vi "Process.vi"(8 "error in":errorcluster, 11 "Instrument UI.Transport":refnum<class "Inst UI.Transport.lvclass">) -> (0 "error out":errorcluster, 3 "Instrument UI.Transport out":refnum<class "Inst UI.Transport.lvclass">)   [LabVIEW 2019, in "Inst UI.Transport.lvclass"]
doc: "---------------------------------------------------------------\nJKI State Machine Objects™\nhttp://jki.net/state-machine-objects/\nCopyright (C) 2005-2015, JKI <info@jki.net>\nALL RIGHTS RESERVEDJKI State Machine Objects (SMO) 1.0.0.5\nJKI - JKI\nCopyright (c) 2016, JKI"
uses:
  Inst UI.Transport.lvclass
  C:/Program Files/National Instruments/LabVIEW 2019/vi.lib/JKI/JKI SMO/SMO/SMO.lvclass
  C:/Program Files/National Instruments/LabVIEW 2019/user.lib/LevyLab/Instrument Framework/Instrument UI/Instrument UI.lvclass
  C:/Program Files/National Instruments/LabVIEW 2019/vi.lib/JKI/JKI SMO/SMO.UI/SMO.UI.lvclass
  Inst.Transport/Typedefs/Inst.Transport.getAll--Cluster.ctl
  Inst.Transport/Inst.Transport.lvclass
  C:/Program Files/National Instruments/LabVIEW 2019/user.lib/LevyLab/Instrument Framework/Instrument/Instrument.lvclass
  Instrument UI.Transport.UI--Cluster.ctl
  Inst.Transport/Typedefs/Inst.Transport.Configuration--Cluster.ctl
  Transport/Typedefs/Lockin_Sweep JSON--Cluster.ctl
  <userlib>/LevyLab/Lockin-Multichannel/Instrument.DAQ/Typedefs/Sweep.Channel--Cluster--Array.ctl
  <userlib>/LevyLab/Lockin-Multichannel/Instrument.DAQ/Typedefs/Sweep.Channel--Cluster.ctl
  <userlib>/LevyLab/Lockin-Multichannel/Instrument.DAQ/Typedefs/Sweep.Pattern--Enum.ctl
  <userlib>/LevyLab/Configuration/Configuration.lvclass
  <userlib>/LevyLab/Instrument Framework/Instrument UI/Instrument UI.lvclass/Instrument UI.ctl
  <vilib>/JKI/JKI SMO/SMO/SMO.lvclass/SMO.ctl
  <userlib>/LevyLab/Configuration/Configuration.lvclass/Configuration.ctl
  2c224a34-a253-4174-b18d-44043a318d1a.vi
  <vilib>/dlg_ctls.llb/Space Constant.vi
  <vilib>/AdvancedString/1D String Array to Delimited String.vi
  <vilib>/JKI/JKI SMO/SMO/Private/ReftoDVR--SMO.vi
  2c224a34-a253-4174-b18d-44043a318d1a.vi/26bc7fe7-399c-42c0-9e9a-60ca208975aa.vi
  2c224a34-a253-4174-b18d-44043a318d1a.vi/9995e869-8f6f-46da-9c29-74663bf4c27c.vi
  <vilib>/Utility/Data Type/Get Type Information.vi
  <vilib>/JDP Science/JSONtext/JSON text to Variant.vi
  <userlib>/LevyLab/Instrument Framework/Instrument/Instrument.lvclass
  <vilib>/JDP Science/JSONtext/LVClass Serializer/JSONtext LVClass Serializer.lvclass
  <userlib>/LevyLab/Instrument Framework/Instrument UI/Instrument UI.lvclass
  <userlib>/LevyLab/Debug/Debug.lvlib
  <vilib>/JKI/JKI SMO/SMO/SMO.lvclass
  <vilib>/JKI/JKI SMO/SMO.UI/SMO.UI.lvclass
  <userlib>/LevyLab/Lockin-Multichannel/Instrument.DAQ/Instrument.DAQ.lvclass
  Transport/Transport.lvclass
panel:
  out "Secret Status":string
  out "State History":string
  in  "STOP":bool
  # "Transport Server"
  # "SMO UI Template"
  # "For instructions on how to use the JKI State Machine Objects, examples and video tutorials, visit:\nhttp://jki.net/state-machine-objects/\n\nJKI State Machine Objects™\nhttp://jki.net/state-machine-objects/\nCopyright (C) 2005-2015, JKI <info@jki.net>\nALL RIGHTS RESERVED"
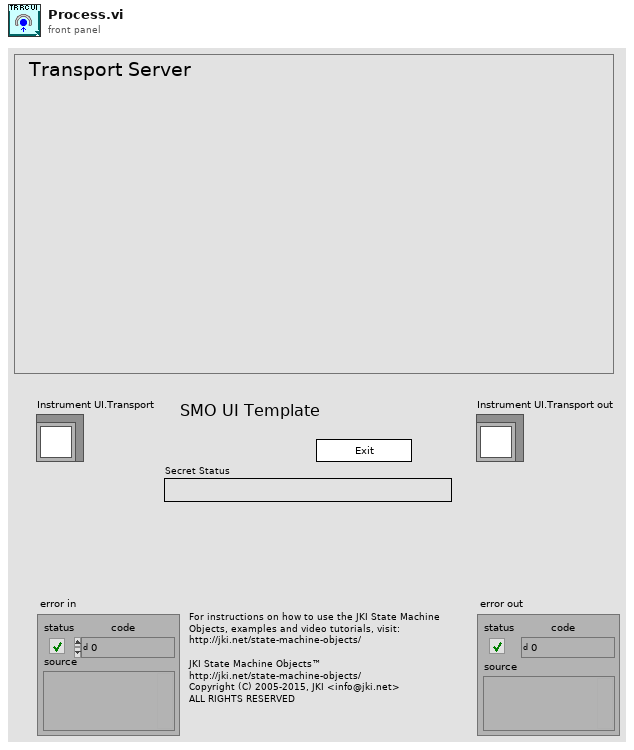
[diagram p1: front panel]
types:
  T1 = enum32{"invalid app kind", "Development System", "Run Time System", "Student Edition", "Embedded LabVIEW", "Evaluation", "Custom"}
  T2 = enum32{"Invalid", "Standard", "Closed", "Hidden", "Minimized", "Maximized"}
  T3 = typedef "Inst.Transport.lvclass/Inst.Transport.Configuration--Cluster.ctl" = cluster{"Folder":string, "Comments":string, "Sweep":T4}
  T4 = typedef "Transport.lvclass/Lockin_Sweep JSON--Cluster.ctl" = cluster{"initialWaitTime":dbl, "sweepTime":dbl, "Return to Start":bool, "sweepChannels":T5, "sweepTables":cluster{"Ch":i32, "Table":dbl[]}[]}
  T5 = typedef "Instrument.Lockin.lvlib/Instrument.DAQ.lvclass/Sweep.Channel--Cluster--Array.ctl" = T6[]
  T6 = typedef "Instrument.Lockin.lvlib/Instrument.DAQ.lvclass/Sweep.Channel--Cluster.ctl" = cluster{"Enable?":bool, "Channel":u16, "Start":dbl, "End":dbl, "Pattern":T7, "Table":dbl[]}
  T7 = typedef "Instrument.Lockin.lvlib/Instrument.DAQ.lvclass/Sweep.Pattern--Enum.ctl" = enum16{"Ramp /", "Ramp /\\", "Smooth Ramp _/", "Smooth Ramp _/\\_", "Table"}
  T8 = typedef "Inst.Transport.lvclass/Inst.Transport.getAll--Cluster.ctl" = cluster{"data":variant}
  T9 = typedef "Inst UI.Transport.lvclass/Instrument UI.Transport.UI--Cluster.ctl" = cluster{"Parameter":dbl, "Parameter 2":string}
  T10 = cluster{"Core":cluster{"Current VI Reference":refnum<vi>, "Close Panel on Exit?":bool, "Last Error":cluster{"error":errorcluster, "previous state":string, "remaining states":string}, "Shutdown?":bool}, "Instrument UI":refnum<class "Inst UI.Transport.lvclass">, "Instrument":refnum<class "Inst.Transport.lvclass">, "Configuration":refnum<class "Configuration.lvclass">, "Config Cluster":T3, "getAll":T8, "UI Cluster":T9, "UI Behavior":string, "wait":u32}
  T11 = cluster{"Current VI Reference":refnum<vi>, "Close Panel on Exit?":bool, "Last Error":cluster{"error":errorcluster, "previous state":string, "remaining states":string}, "Shutdown?":bool}
  T12 = typedef "Debug.lvlib/Attribute.Debug.lvclass/DebugBehavior.ctl" = enum16{"Normal", "Debug"}
  T13 = typedef "SMO.lvclass/Protected Events.ctl" = cluster{"StopProcesses":refnum<user-event>, "AbortProcesses":refnum<user-event>, "Config Changed":refnum<user-event>, "Dependency":refnum<user-event>}
  T14 = typedef "Instrument.lvlib/Instrument.lvclass/PublicEvents--Cluster.ctl" = cluster{"MessageFromProcess":refnum<user-event>}
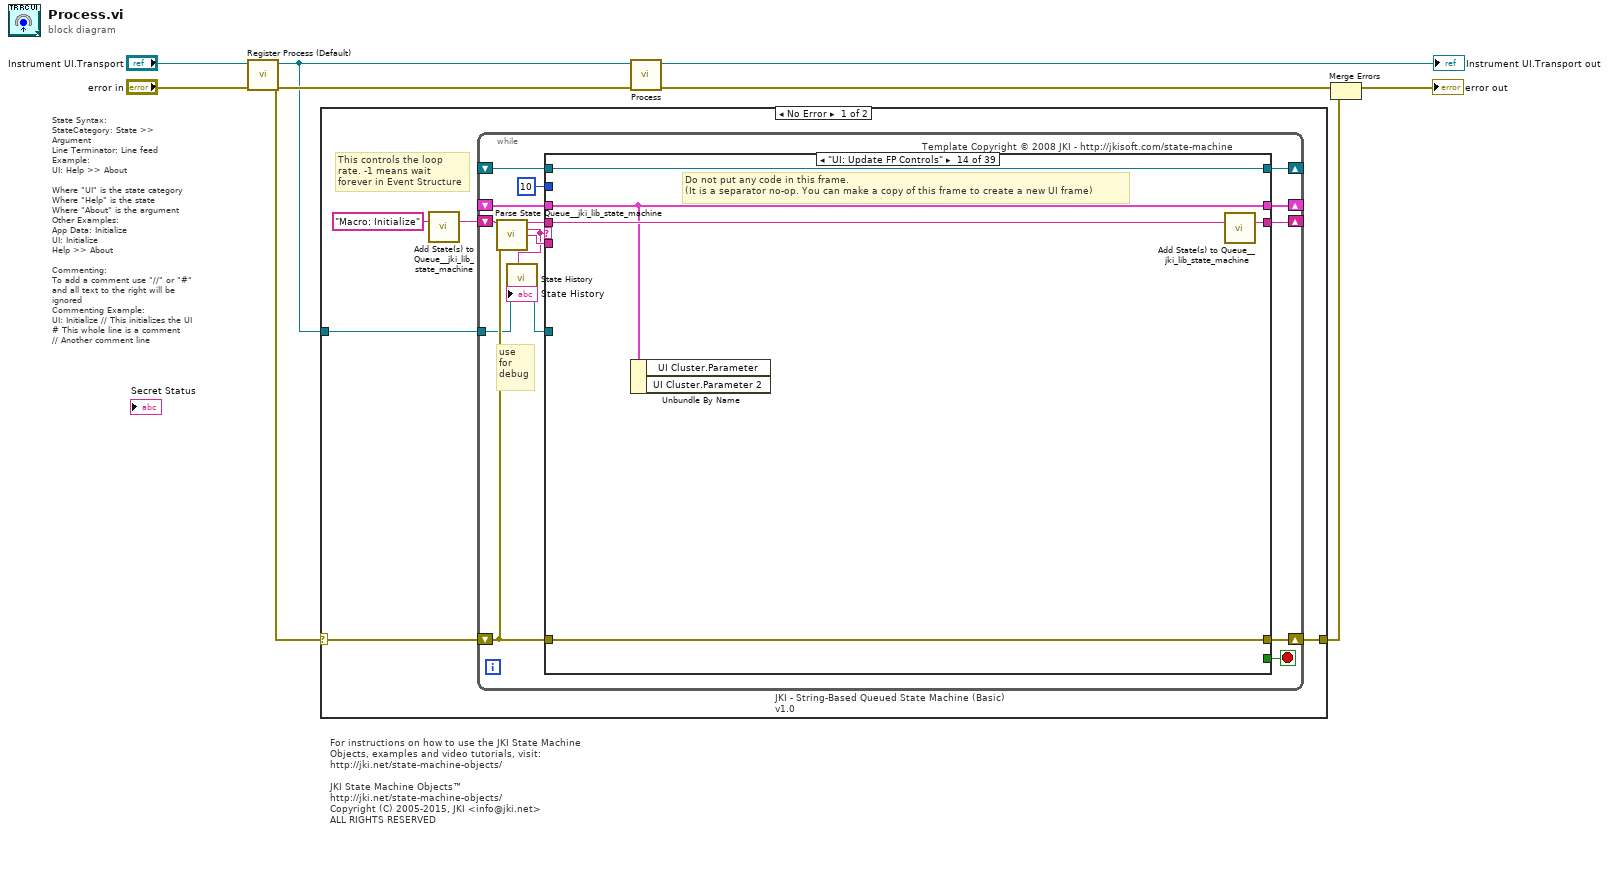
[diagram p0: block diagram]
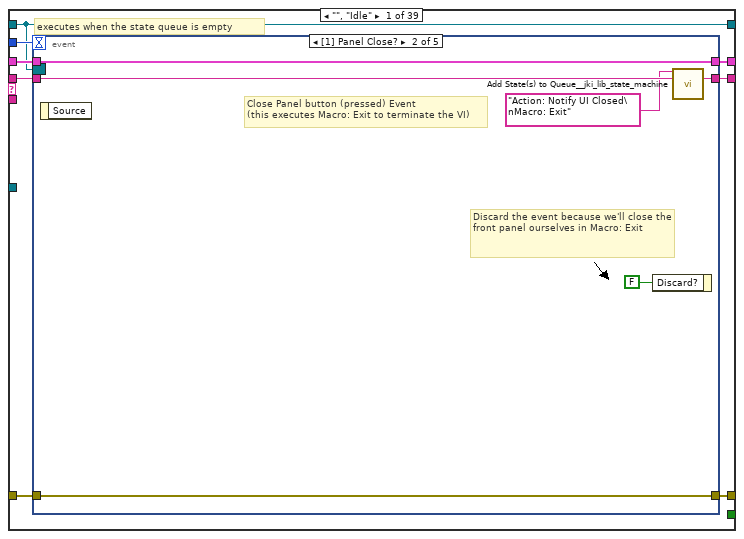
[diagram p2: hidden frame]
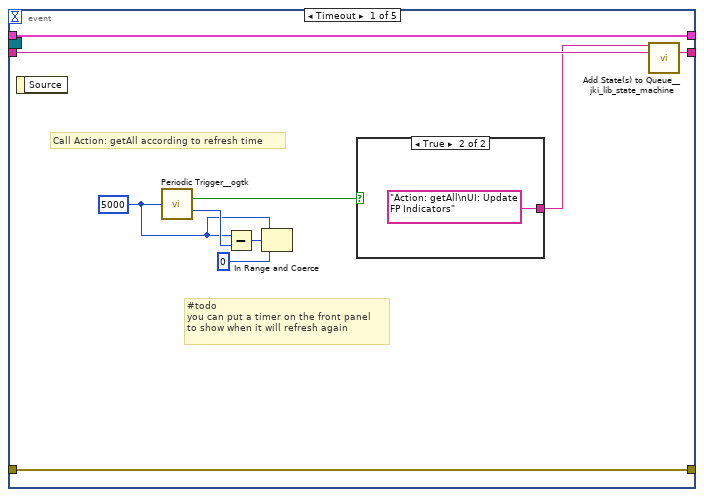
[diagram p3: hidden frame]
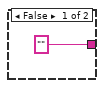
[diagram p4: hidden frame]
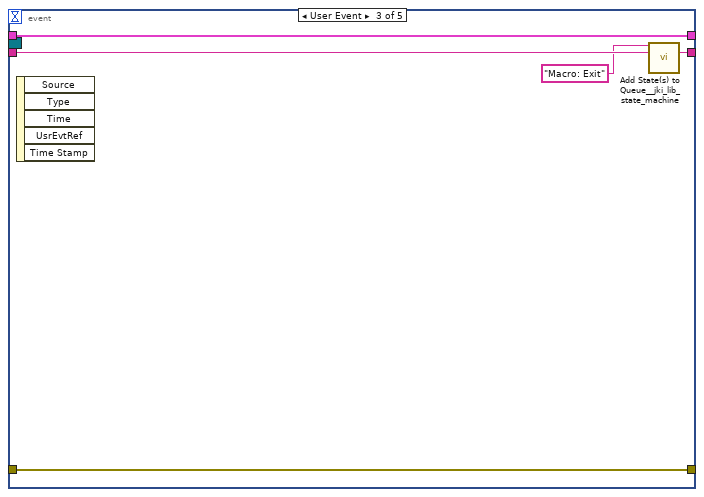
[diagram p5: hidden frame]
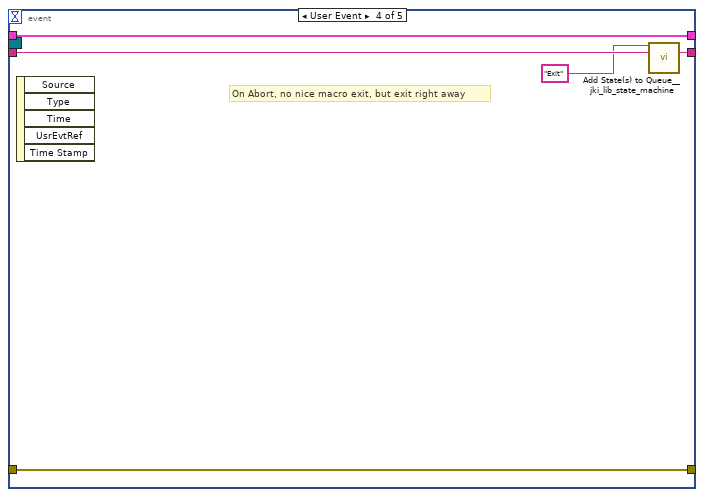
[diagram p6: hidden frame]
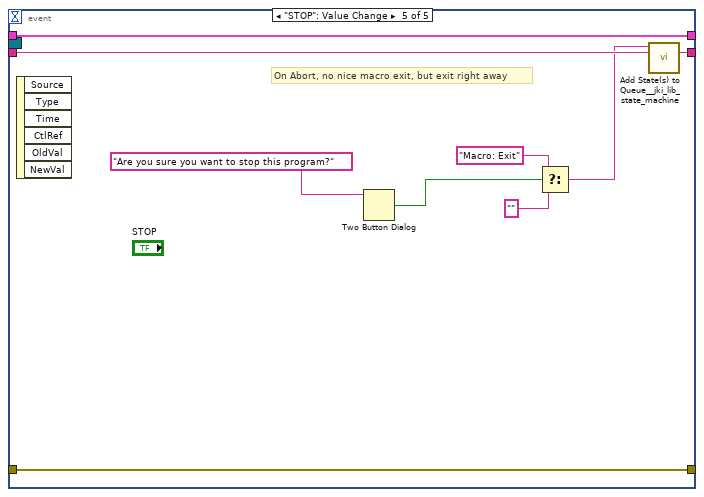
[diagram p7: hidden frame]
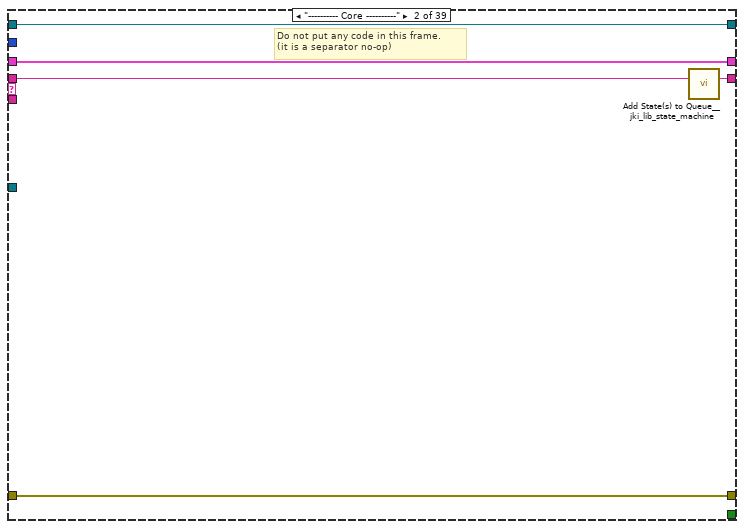
[diagram p8: hidden frame]
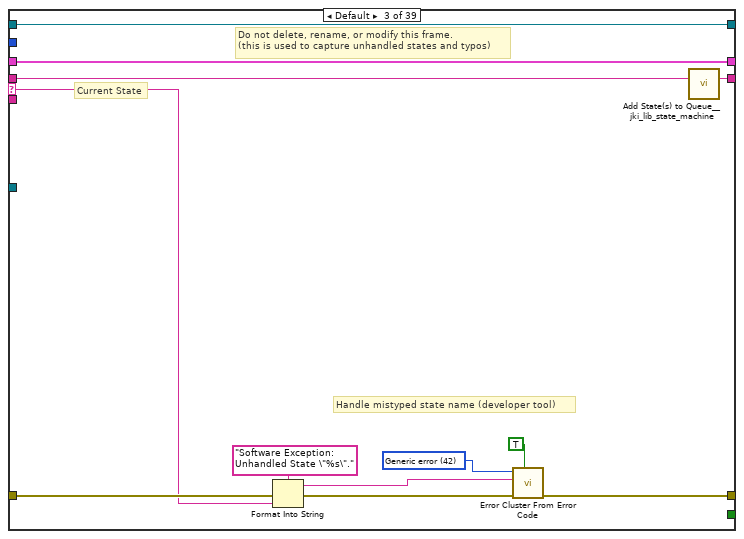
[diagram p9: hidden frame]
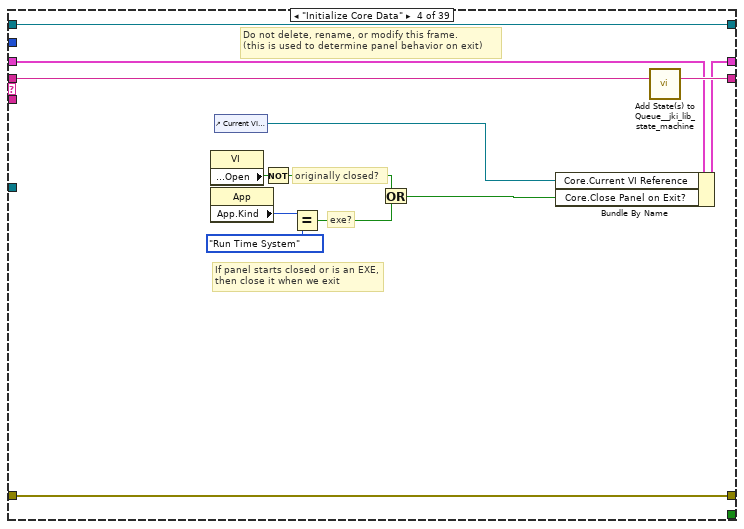
[diagram p10: hidden frame]
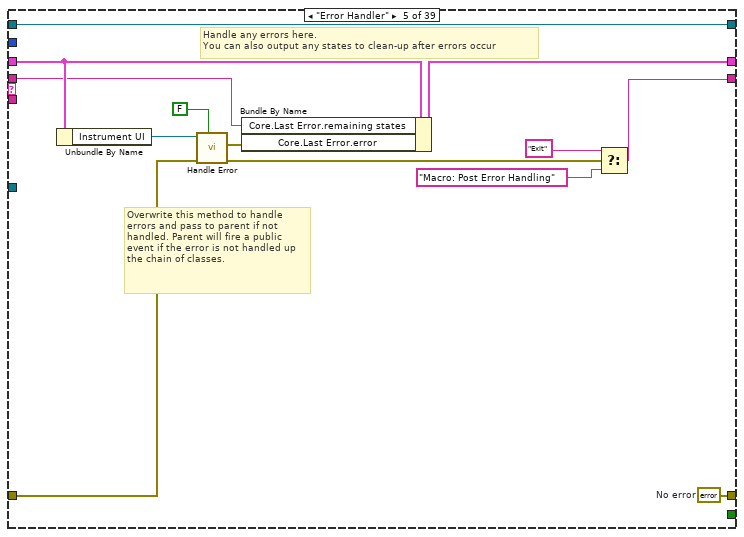
[diagram p11: hidden frame]
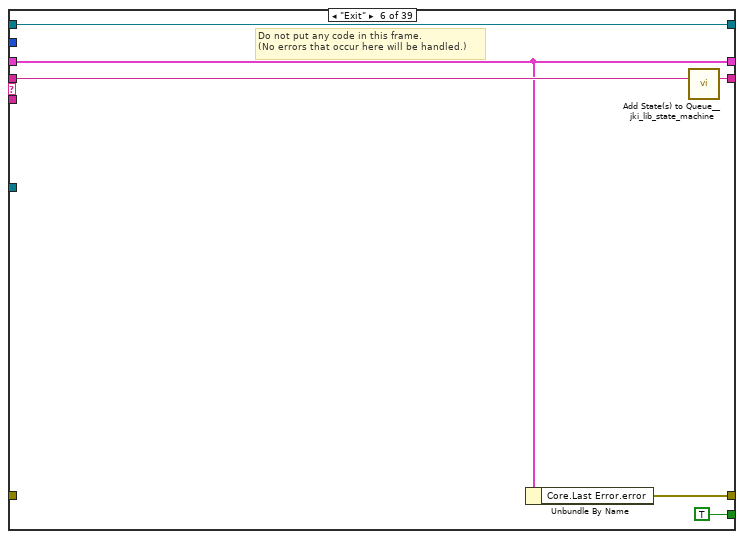
[diagram p12: hidden frame]
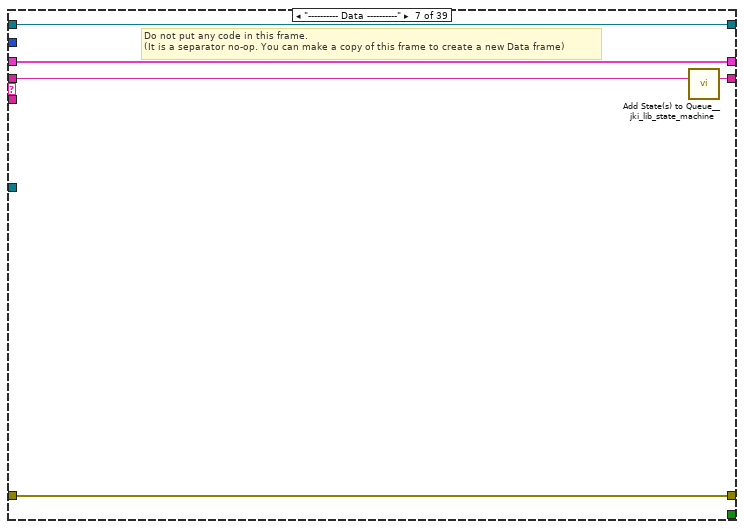
[diagram p13: hidden frame]
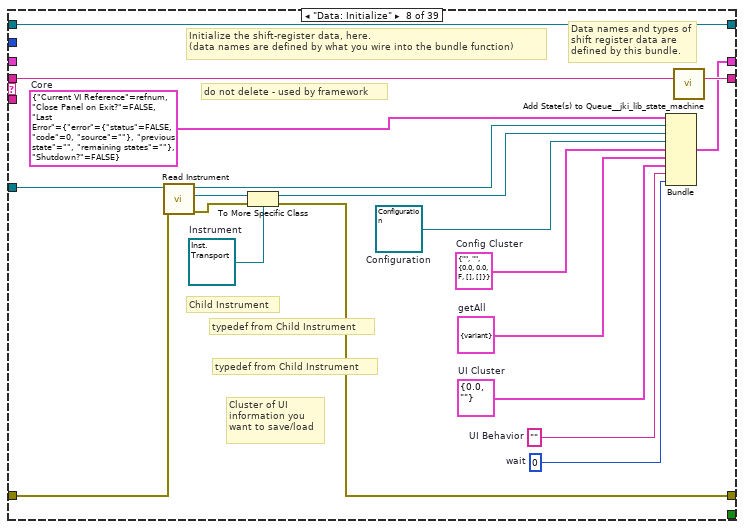
[diagram p14: hidden frame]
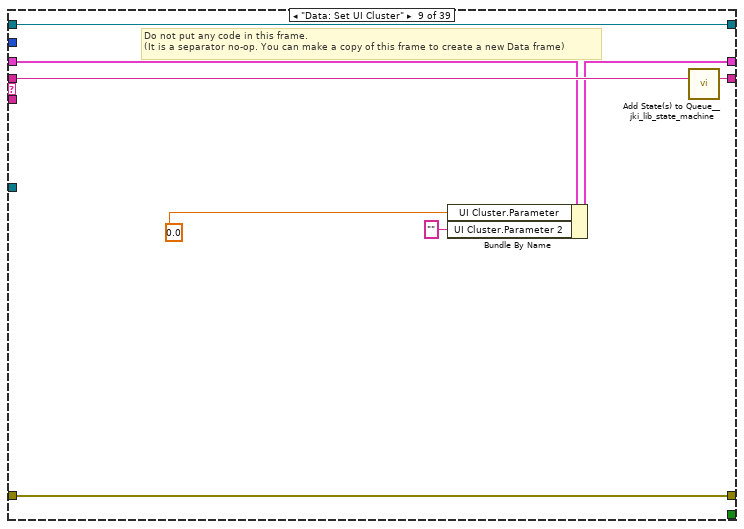
[diagram p15: hidden frame]
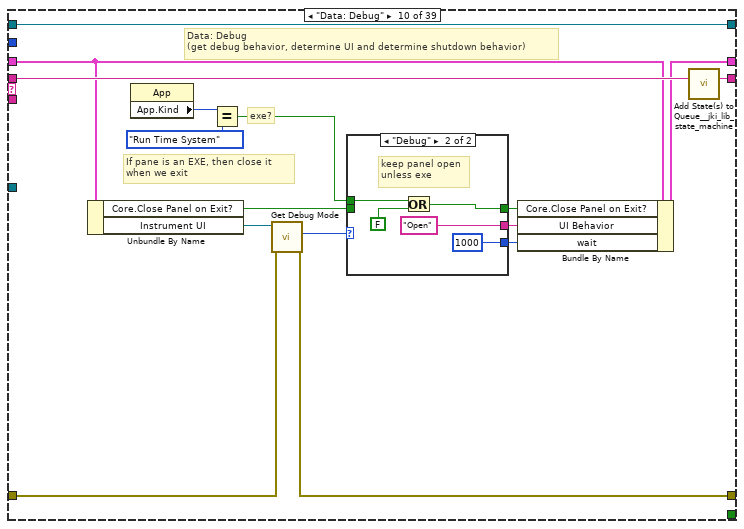
[diagram p16: hidden frame]
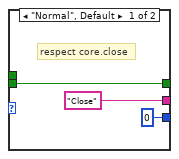
[diagram p17: hidden frame]
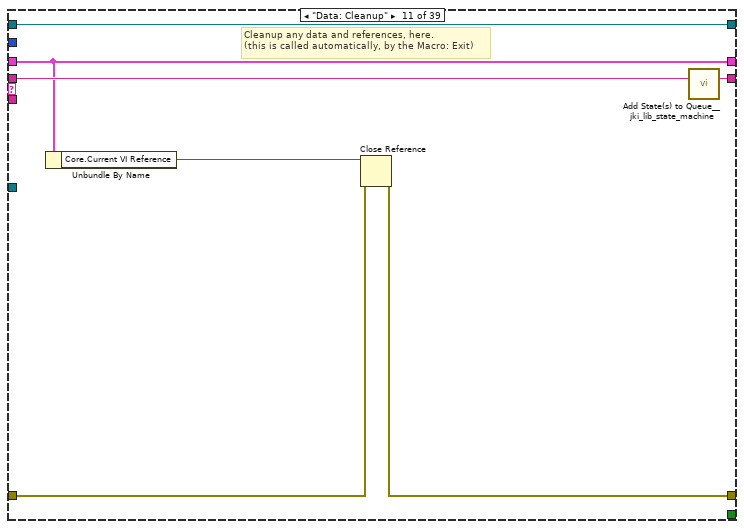
[diagram p18: hidden frame]
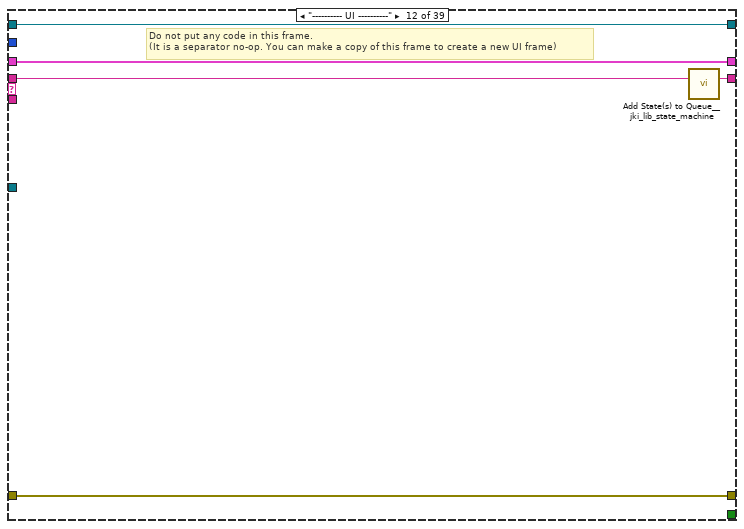
[diagram p19: hidden frame]
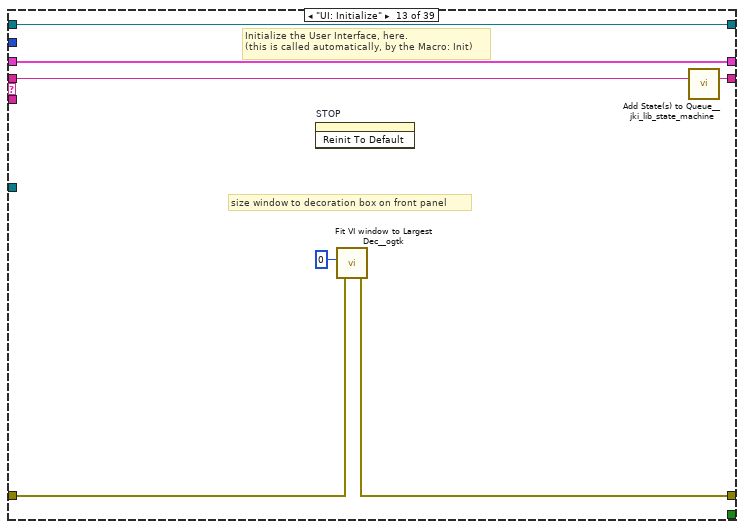
[diagram p20: hidden frame]
diagram:
  # "State Syntax:\nStateCategory: State >> Argument\nLine Terminator: Line feed\nExample:\nUI: Help >> About\n\nWhere \"UI\" is the state category\nWhere \"Help\" is the state\nWhere \"About\" is the argument\nOther Examples:\nApp Data: Initialize\nUI: Initialize\nHelp >> About\n\nCommenting:\nTo add a comment use \"//\" or \"#\" and all text to the right will be ignored\nCommenting Example:\nUI: Initialize // This initializes the UI\n# This whole line is a comment\n// Another comment line"
  # "For instructions on how to use the JKI State Machine Objects, examples and video tutorials, visit:\nhttp://jki.net/state-machine-objects/\n\nJKI State Machine Objects™\nhttp://jki.net/state-machine-objects/\nCopyright (C) 2005-2015, JKI <info@jki.net>\nALL RIGHTS RESERVED"
  n1 = call <vilib>:"Register Process (Default).vi"("error in (no error)"="error in", "SMO"="Instrument UI.Transport") -> ("error out"=w5:errorcluster, "SelfRef"=w4:refnum<class "Inst UI.Transport.lvclass">)  [unwired: 8 in]
  n2 = case shown="No Error" w5 {
    selector: w5 -> [w10 w459]
    tunnel: w4 -> [w11 _]
    tunnel: [w9 w459] -> w1
    frame No Error {
      # "This controls the loop rate. -1 means wait forever in Event Structure"
      n3 = call <vilib>:"Add State(s) to Queue__jki_lib_state_machine.vi"("State(s) in (\"\")"="Macro: Initialize") -> ("States Out"=w13:string)  [unwired: 14 in]
      n4 = while "JKI - String-Based Queued State Machine (Basic) v1.0" {
        shift-right: [w23] -> _
        shift-left: _ -> [w22]
        shift-right: [w26] -> w9
        shift-left: w10 -> [w18]
        shift-right: [w25] -> _
        shift-left: w13 -> [w27]
        tunnel: w11 -> [w14]
        shift-right: [w20] -> _
        shift-left: _ -> [w19]
        stop <- w24 stop-if-true
        # "use\nfor\ndebug"
        # "Template Copyright © 2008 JKI - http://jkisoft.com/state-machine"
        n5 = call <vilib>:"Parse State Queue__jki_lib_state_machine.vi"("State Queue"=w27, "Error In (no error)"=w18) -> ("Remaining States"=w29:string, "Current State"=w17:string, "Arguments"=w28:string)  [unwired: 11 in]
        n6 = call <userlib>:"State History.vi"("Current State"=w17, "SMO"=w14) -> ("SMO"=w15:refnum<class "Inst UI.Transport.lvclass">, "History"=→"State History":string)  [unwired: 8 in]
        n7 = case shown="\"UI: Update FP Controls\"" w17 {
          selector: w17 -> [_ _ w81 _ _ _ _ _ _ _ _ _ _ _ _ _ _ _ _ _ _ _ _ _ _ _ _ _ _ _ _ _ _ _ _ _ _ _ _]
          tunnel: w29 -> [w37 w79 w85 w104 w108 w123 w128 w147 w155 w171 w186 w191 w198 w203 w208 w215 w231 w263 w272 w284 w294 w300 w308 w323 w328 w339 w346 w351 w364 w370 w375 w390 w398 w410 w417 w424 w438 w448 w458]
          tunnel: w28 -> [_ _ _ _ _ _ _ _ _ _ _ _ _ _ _ w209 w225 _ _ _ _ _ _ _ _ _ _ _ _ _ _ _ _ _ _ _ _ _ _]
          tunnel: w22 -> [w35 w76 w83 w95 w111 w119 w125 _ w151 w158 w180 w188 w196 w199 w204 w213 w227 w260 w269 w274 w291 w297 w302 w312 w325 w336 w341 w348 w362 w368 w372 w383 w395 w401 w413 w418 w433 w442 w450]
          tunnel: [w34 w77 w87 w101 w113 w118 w126 w129 w153 w157 w182 w189 w193 w201 w205 w210 w228 w261 w264 w282 w292 w298 w306 w321 w326 w330 w342 w349 w357 w365 w373 w376 w393 w402 w414 w419 w431 w445 w455] -> w26
          tunnel: [w36 w78 w84 w103 w105 w122 w127 w146 w154 w170 w185 w190 w197 w202 w207 w214 w230 w262 w271 w283 w293 w299 w307 w322 w327 w338 w345 w350 w363 w369 w374 w389 w397 w409 w416 w423 w437 w447 w457] -> w25
          tunnel: [_ _ _ _ _ TRUE _ _ _ _ _ _ _ _ _ _ _ _ _ _ _ _ _ _ _ _ _ _ _ _ _ _ _ _ _ _ _ _ _] -> w24
          tunnel: [w32 w76 w83 w102 w110 w119 w125 w145 w150 w159 w180 w188 w196 w199 w204 w213 w227 w260 w269 w275 w291 w297 w302 w312 w325 w336 w341 w348 w362 w368 w372 w387 w395 w399 w412 w418 w434 w443 w452] -> w23
          tunnel: 10 ("Timeout") -> [w31 _ _ _ _ _ _ _ _ _ _ _ _ _ _ _ _ _ _ _ _ _ _ _ _ _ _ _ _ _ _ _ _ _ _ _ _ _ _]
          tunnel: w15 -> [_ _ _ _ _ _ _ w134 _ _ _ _ _ _ _ _ _ _ _ _ _ _ _ _ _ _ _ _ _ _ _ _ _ _ _ _ _ _ _]
          tunnel: [w30 w75 w80 w92 w117 w120 w124 w144 w152 w169 w181 w187 w195 w200 w206 w212 w224 w259 w270 w281 w290 w296 w305 w317 w324 w337 w344 w347 w361 w367 w371 w388 w396 w408 w415 w422 w436 w446 w456] -> w20
          tunnel: w19 -> [w30 w75 w80 w92 w117 w120 w124 w144 w152 w169 w181 w187 w195 w200 w206 w212 w224 w259 w270 w281 w290 w296 w305 w317 w324 w337 w344 w347 _ w367 w371 w388 w396 w408 w415 w422 w436 w446 w456]
          tunnel: w18 -> [w33 w77 w86 w101 w107 _ w126 w133 w153 w156 w183 w189 w194 w201 w205 w211 w229 w261 w264 w282 w292 w298 w306 w321 w326 w331 w343 w349 w359 w366 w373 w385 w391 w403 w414 w420 w425 w439 w451]
          frame "", "Idle" {
            # "executes when the state queue is empty"
            n8 = event shown="[1] Panel Close?" {
              selector: w30 -> [_ _ _ _ _]
              dyn-events: _ -> [_ _ _ _ _]
              timeout: w31 -> [_ _ _ _ _]
              tunnel: w37 -> [w47 w55 w60 w65 w74]
              tunnel: [w46 w54 w59 w64 w73] -> w36
              tunnel: w35 -> [w44 w51 w57 w62 w71]
              tunnel: [w45 w50 w58 w63 w72] -> w34
              tunnel: w33 -> [w45 w50 w58 w63 w72]
              tunnel: [w44 w51 w57 w62 w71] -> w32
              event Timeout {
                w39 = u32 5000 ("time (ms)")
                # "#todo\nyou can put a timer on the front panel\nto show when it will refresh again"
                # "Call Action: getAll according to refresh time"
                n9 = event-data() -> ()  [unwired: 1 in, 1 out]
                n10 = call <userlib>:"Periodic Trigger__ogtk.vi"("time (ms)"=w39) -> ("Triggered"=w42:bool, "timer value"=w41:u32)  [unwired: 12 in, 1 out]
                n11 = Subtract(x=w39, y=w41) -> (x-y=w40:u32)
                n12 = In Range and Coerce(upper limit=w39, x=w40, lower limit=u32 0) -> ()  [unwired: 2 out]
                n13 = case shown="True" w42 {
                  tunnel: ["" ("State(s) in Front (\"\")") "Action: getAll\nUI: Update FP Indicators" ("State(s) in Front (\"\")")] -> w43
                  frame False {
                  }
                  frame True {
                  }
                }
                n14 = call <vilib>:"Add State(s) to Queue__jki_lib_state_machine.vi"("State(s) in Front (\"\")"=w43, "State(s) in (\"\")"=w47) -> ("States Out"=w46:string)  [unwired: 13 in]
              }
              event Panel Close? {
                # "Discard the event because we'll close the front panel ourselves in Macro: Exit"
                # "Close Panel button (pressed) Event\n(this executes Macro: Exit to terminate the VI)"
                n15 = event-data() -> ()  [unwired: 1 in, 1 out]
                n16 = event-data("Discard?"=FALSE) -> ()  [unwired: 1 in, 1 out]
                n17 = call <vilib>:"Add State(s) to Queue__jki_lib_state_machine.vi"("State(s) in Front (\"\")"="Action: Notify UI Closed\nMacro: Exit", "State(s) in (\"\")"=w55) -> ("States Out"=w54:string)  [unwired: 13 in]
              }
              event User Event {
                n18 = event-data() -> ()  [unwired: 1 in, 5 out]
                n19 = call <vilib>:"Add State(s) to Queue__jki_lib_state_machine.vi"("State(s) in Front (\"\")"="Macro: Exit", "State(s) in (\"\")"=w60) -> ("States Out"=w59:string)  [unwired: 13 in]
              }
              event User Event {
                # "On Abort, no nice macro exit, but exit right away"
                n20 = event-data() -> ()  [unwired: 1 in, 5 out]
                n21 = call <vilib>:"Add State(s) to Queue__jki_lib_state_machine.vi"("State(s) in Front (\"\")"="Exit", "State(s) in (\"\")"=w65) -> ("States Out"=w64:string)  [unwired: 13 in]
              }
              event "STOP": Value Change {
                # "On Abort, no nice macro exit, but exit right away"
                n22 = event-data() -> ()  [unwired: 1 in, 6 out]
                n23 = Two Button Dialog(message="Are you sure you want to stop this program?") -> (T button?=w70:bool)  [unwired: 2 in]
                n24 = Select(t="Macro: Exit", s=w70, f="") -> (s? t:f=w66:string)
                n25 = call <vilib>:"Add State(s) to Queue__jki_lib_state_machine.vi"("State(s) in Front (\"\")"=w66, "State(s) in (\"\")"=w74) -> ("States Out"=w73:string)  [unwired: 13 in]
              }
            }
          }
          frame "---------- Core ----------" {
            # "Do not put any code in this frame.\n(it is a separator no-op)"
            n26 = call <vilib>:"Add State(s) to Queue__jki_lib_state_machine.vi"("State(s) in (\"\")"=w79) -> ("States Out"=w78:string)  [unwired: 14 in]
          }
          frame Default {
            w90 = 42 items=["No error", "Argument error", "Memory is full", "Out of zone", "End of file", "File already open", "Generic file I/O error", "File not found", "File permission error", "Disk is full", "Duplicate path", "Too many files open", "System feature not enabled", "Resource file not found", "Cannot add resource", "Resource not found", "Image not found", "Image memory error", "Pen does not exist", "Config type invalid", "Config token not found", "Config parse error", "Config memory error", "Bad external code format", "Bad external code offset", "External code not present", "Null window", "Destroy window error", "Null menu", "Print aborted", "Bad print record", "Print driver error", "Windows error during printing", "Memory error during printing", "Print dialog error", "Generic print error", "Invalid device refnum", "Device not found", "Device parameter error", "Device unit error", "Cannot open device", "Device call aborted", "Generic error", "Cancelled by user", "Object ID too low", "Object ID too high", "Object not in heap", "Unknown heap", "Unknown object (invalid DefProc)", "Unknown object (DefProc not in table)", "Message out of range", "Invalid (null) method", "Unknown message", "Manager call not supported", "Bad address", "Network operation in progress", "Network operation timed out", "Connection is busy", "Network attribute not supported", "Network error", "Address in use", "System out of memory", "Connection aborted", "Connection refused", "Not connected", "Already connected", "Connection closed", "Initialization error (interapplication manager)", "Bad occurrence", "Wait on unbound occurrence handler", "Occurrence queue overflow", "Datalog type conflict", "Unused", "Unrecognized type (interapplication manager)", "Memory corrupt", "Failed to make temporary DLL", "Old CIN version", "Drag socket not found", "Failed to load drop-object", "Failed to register OLE object", "Failed to release OLE object", "Format specifier type mismatch", "Unknown format specifier", "Too few format specifiers", "Too many format specifiers", "Scan failed", "Newer CIN version", "Error converting to variant", "Runtime menu error", "Password tampered", "Variant attribute not found", "Incompatible variant data type", "Event data is not available", "Event Store is not present", "Occurrence is not found", "Event Queue is not created", "Event info is not available", "Refnum passed is NULL", "Error retrieving Class GUID", "Error retrieving CoClass GUID", "Error retrieving TypeLib GUID.", "Bad built application magic bytes.", "Specific driver is different from the specific driver associated with the Logical Name.", "There is no session opened to the class driver.", "Max Error", "MAX - Error with config objects", "MAX - Error loading configuration", "MAX - Group not supported"]
            # "Current State"
            # "Do not delete, rename, or modify this frame.\n(this is used to capture unhandled states and typos)"
            # "Handle mistyped state name (developer tool)"
            n27 = Format Into String(format string="Software Exception: Unhandled State \"%s\"." ("message"), error in=w86, w81) -> (resulting string=w89:string, error out=w88:errorcluster)  [unwired: 1 in]
            n28 = call <vilib>:"Error Cluster From Error Code.vi"("show call chain? (False)"=TRUE, "error in (no error)"=w88, "error message (\"\")"=w89, "error code (0)"=w90) -> ("error out"=w87:errorcluster)  [unwired: 5 in]
            n29 = call <vilib>:"Add State(s) to Queue__jki_lib_state_machine.vi"("State(s) in (\"\")"=w85) -> ("States Out"=w84:string)  [unwired: 14 in]
          }
          frame "Initialize Core Data" {
            # "Do not delete, rename, or modify this frame.\n(this is used to determine panel behavior on exit)"
            # "originally closed?"
            # "exe?"
            # "If panel starts closed or is an EXE, then close it when we exit"
            n30 = property class="VI"() -> ("Front Panel.Open"=w100:bool)  [unwired: 2 in, 2 out]
            n31 = property class="App"() -> ("App.Kind"=w99:T1)  [unwired: 2 in, 2 out]
            n32 = control-ref of="Current VI Reference"() -> (w93:refnum<vi>)
            n33 = Not(x=w100) -> (.not. x?=w97:bool)
            n34 = Equal?(x=w99, y=T1."Run Time System" ("Application:Kind")) -> (x = y?=w96:bool)
            n35 = Or(x=w97, y=w96) -> (x .or. y?=w94:bool)
            n36 = Bundle By Name(cluster=w95, "Core.Current VI Reference"=w93, "Core.Close Panel on Exit?"=w94) -> (w102:T10)
            n37 = call <vilib>:"Add State(s) to Queue__jki_lib_state_machine.vi"("State(s) in (\"\")"=w104) -> ("States Out"=w103:string)  [unwired: 14 in]
          }
          frame "Error Handler" {
            w113 = errorcluster {"status"=FALSE, "code"=0, "source"=""}  # No error
            # "Overwrite this method to handle errors and pass to parent if not handled. Parent will fire a public event if the error is not handled up the chain of classes."
            # "Handle any errors here.\nYou can also output any states to clean-up after errors occur"
            n38 = Unbundle By Name(w111) -> ("Instrument UI"=w116:refnum<class "Inst UI.Transport.lvclass">)
            n39 = call-dynamic "Handle Error.vi"("Stop on Unhandled Error (T)"=FALSE, "error in"=w107, "SMO"=w116) -> ("handling error"=w114:errorcluster, "Unhandled error"=w112:errorcluster)  [unwired: 6 in, 1 out]
            n40 = Bundle By Name(cluster=w111, "Core.Last Error.remaining states"=w108, "Core.Last Error.error"=w112) -> (w110:T10)
            n41 = Select(t="Exit", s=w114, f="Macro: Post Error Handling") -> (s? t:f=w105:string)
          }
          frame "Exit" {
            # "Do not put any code in this frame.\n(No errors that occur here will be handled.)"
            n42 = Unbundle By Name(w119) -> ("Core.Last Error.error"=w118:errorcluster)
            n43 = call <vilib>:"Add State(s) to Queue__jki_lib_state_machine.vi"("State(s) in (\"\")"=w123) -> ("States Out"=w122:string)  [unwired: 14 in]
          }
          frame "---------- Data ----------" {
            # "Do not put any code in this frame.\n(It is a separator no-op. You can make a copy of this frame to create a new Data frame)"
            n44 = call <vilib>:"Add State(s) to Queue__jki_lib_state_machine.vi"("State(s) in (\"\")"=w128) -> ("States Out"=w127:string)  [unwired: 14 in]
          }
          frame "Data: Initialize" {
            w130 = u32 0  # wait
            w131 = ""  # UI Behavior
            w135 = refnum<class "Configuration.lvclass"> refnum  # Configuration
            w137 = T3 {"Folder"="", "Comments"="", "Sweep"={"initialWaitTime"=0.0, "sweepTime"=0.0, "Return to Start"=FALSE, "sweepChannels"=[], "sweepTables"=[]}}  # Config Cluster
            w139 = T9 {"Parameter"=0.0, "Parameter 2"=""}  # UI Cluster
            w141 = refnum<class "Inst.Transport.lvclass"> refnum  # Instrument
            w142 = T8 {"data"=variant(string "")}  # getAll
            w143 = T11 {"Current VI Reference"=refnum, "Close Panel on Exit?"=FALSE, "Last Error"={"error"={"status"=FALSE, "code"=0, "source"=""}, "previous state"="", "remaining states"=""}, "Shutdown?"=FALSE}  # Core
            # "typedef from Child Instrument"
            # "Cluster of UI\ninformation you\nwant to save/load"
            # "Child Instrument"
            # "typedef from Child Instrument"
            # "do not delete - used by framework"
            # "Data names and types of shift register data are defined by this bundle."
            # "Initialize the shift-register data, here.\n(data names are defined by what you wire into the bundle function)"
            n45 = call <userlib>:"Read Instrument.vi"("error in (no error)"=w133, "Instrument UI in"=w134) -> ("error out"=w138:errorcluster, "Instrument"=w140:refnum<class "Instrument.lvclass">, "Instrument UI"=w132:refnum<class "Inst UI.Transport.lvclass">)  [unwired: 7 in]
            n46 = To More Specific Class(target class=w141, reference=w140, error in=w138) -> (specific class reference=w136:refnum<class "Inst.Transport.lvclass">, error out=w129:errorcluster)
            n47 = Bundle("Core"=w143, "Instrument UI"=w132, "Instrument"=w136, "Configuration"=w135, "Config Cluster"=w137, "getAll"=w142, "UI Cluster"=w139, "UI Behavior"=w131, "wait"=w130) -> (w145:T10)  [unwired: 1 in]
            n48 = call <vilib>:"Add State(s) to Queue__jki_lib_state_machine.vi"("State(s) in (\"\")"=w147) -> ("States Out"=w146:string)  [unwired: 14 in]
          }
          frame "Data: Set UI Cluster" {
            # "Do not put any code in this frame.\n(It is a separator no-op. You can make a copy of this frame to create a new Data frame)"
            n49 = Bundle By Name(cluster=w151, "UI Cluster.Parameter"=0.0, "UI Cluster.Parameter 2"="") -> (w150:T10)
            n50 = call <vilib>:"Add State(s) to Queue__jki_lib_state_machine.vi"("State(s) in (\"\")"=w155) -> ("States Out"=w154:string)  [unwired: 14 in]
          }
          frame "Data: Debug" {
            # "exe?"
            # "If pane is an EXE, then close it when we exit"
            # "Data: Debug\n(get debug behavior, determine UI and determine shutdown behavior)"
            n51 = Unbundle By Name(w158) -> ("Core.Close Panel on Exit?"=w161:bool, "Instrument UI"=w168:refnum<class "Inst UI.Transport.lvclass">)
            n52 = property class="App"() -> ("App.Kind"=w164:T1)  [unwired: 2 in, 2 out]
            n53 = Equal?(x=w164, y=T1."Run Time System" ("Application:Kind")) -> (x = y?=w160:bool)
            n54 = call <userlib>:"Get Debug Mode.vi"("error in (no error)"=w156, "SMO"=w168) -> ("error out"=w157:errorcluster, "Behavior"=w167:T12)  [unwired: 7 in, 1 out]
            n55 = case shown="\"Debug\"" w167 {
              tunnel: ["Close" "Open"] -> w166
              tunnel: [u32 0 ("wait") u32 1000 ("wait")] -> w165
              tunnel: [w172 w175] -> w162
              tunnel: w161 -> [w172 _]
              tunnel: w160 -> [_ w177]
              frame "Normal", Default {
                # "respect core.close"
              }
              frame "Debug" {
                # "keep panel open\nunless exe"
                n56 = Or(x=w177, y=FALSE) -> (x .or. y?=w175:bool)
              }
            }
            n57 = Bundle By Name(cluster=w158, "Core.Close Panel on Exit?"=w162, "UI Behavior"=w166, "wait"=w165) -> (w159:T10)
            n58 = call <vilib>:"Add State(s) to Queue__jki_lib_state_machine.vi"("State(s) in (\"\")"=w171) -> ("States Out"=w170:string)  [unwired: 14 in]
          }
          frame "Data: Cleanup" {
            # "Cleanup any data and references, here.\n(this is called automatically, by the Macro: Exit)"
            n59 = Unbundle By Name(w180) -> ("Core.Current VI Reference"=w184:refnum<vi>)
            n60 = Close Reference(reference=w184, error in (no error)=w183) -> (error out=w182:errorcluster)
            n61 = call <vilib>:"Add State(s) to Queue__jki_lib_state_machine.vi"("State(s) in (\"\")"=w186) -> ("States Out"=w185:string)  [unwired: 14 in]
          }
          frame "---------- UI ----------" {
            # "Do not put any code in this frame.\n(It is a separator no-op. You can make a copy of this frame to create a new UI frame)"
            n62 = call <vilib>:"Add State(s) to Queue__jki_lib_state_machine.vi"("State(s) in (\"\")"=w191) -> ("States Out"=w190:string)  [unwired: 14 in]
          }
          frame "UI: Initialize" {
            # "size window to decoration box on front panel"
            # "Initialize the User Interface, here.\n(this is called automatically, by the Macro: Init)"
            n63 = invoke on="STOP" class="Bool (strict)" method="Reinit To Default"() -> ()  [unwired: 3 in, 3 out]
            n64 = call <userlib>:"Fit VI window to Largest Dec__ogtk.vi"("error in (no error)"=w194, "border spacing (2 px)"=0) -> ("error out"=w193:errorcluster)  [unwired: 4 in, 1 out]
            n65 = call <vilib>:"Add State(s) to Queue__jki_lib_state_machine.vi"("State(s) in (\"\")"=w198) -> ("States Out"=w197:string)  [unwired: 14 in]
          }
          frame "UI: Update FP Controls" {
            # "Do not put any code in this frame.\n(It is a separator no-op. You can make a copy of this frame to create a new UI frame)"
            n66 = Unbundle By Name(w199) -> ()  [unwired: 2 out]
            n67 = call <vilib>:"Add State(s) to Queue__jki_lib_state_machine.vi"("State(s) in (\"\")"=w203) -> ("States Out"=w202:string)  [unwired: 14 in]
          }
          frame "UI: Update FP Indicators" {
            n68 = Unbundle By Name(w204) -> ()  [unwired: 1 out]
            n69 = call <vilib>:"Add State(s) to Queue__jki_lib_state_machine.vi"("State(s) in (\"\")"=w208) -> ("States Out"=w207:string)  [unwired: 14 in]
          }
          frame "UI: Cursor Set" {
            # "Argument"
            # "Initialize the User Interface, here.\n(this is called automatically, by the Macro: Init)"
            n70 = disable-structure shown="Default" {
              disable-tunnel: w211 -> [w216 w219]
              disable-tunnel: [w216 w218] -> w210
              disable-tunnel: w209 -> [_ w217]
              frame condition #0 {
              }
              frame condition #1 (active) {
                n71 = case shown="\"Busy\"" w217 {
                  tunnel: w219 -> [w221 w223]
                  tunnel: [w220 w222] -> w218
                  frame "Idle", Default {
                    n72 = call <vilib>:"Unset Busy.vi"("error in (no error)"=w221) -> ("error out"=w220:errorcluster)  [unwired: 10 in]
                  }
                  frame "Busy" {
                    n73 = call <vilib>:"Set Busy.vi"("error in (no error)"=w223) -> ("error out"=w222:errorcluster)  [unwired: 9 in, 1 out]
                  }
                }
              }
            }
            n74 = call <vilib>:"Add State(s) to Queue__jki_lib_state_machine.vi"("State(s) in (\"\")"=w215) -> ("States Out"=w214:string)  [unwired: 14 in]
          }
          frame "UI: Front Panel State" {
            # "Argument"
            # "Set Front Panel Open or Closed\n(Usage: \"UI: Front Panel State >> Open|Close\")"
            n75 = Unbundle By Name(w227) -> ("Core.Current VI Reference"=w226:refnum<vi>)
            n76 = disable-structure shown="Default" {
              disable-tunnel: w229 -> [w235 w258]
              disable-tunnel: [w234 w258] -> w228
              disable-tunnel: w226 -> [w233 _]
              disable-tunnel: w225 -> [w232 _]
              frame condition #0 (active) {
                n77 = case shown="\"Close\"" w232 {
                  tunnel: w235 -> [w239 w252]
                  tunnel: [w241 w253] -> w234
                  tunnel: w233 -> [w240 w250]
                  frame "Open", Default {
                    n78 = property class="VI"(reference=w240, error in=w239) -> (reference out=w237:refnum<vi>, error out=w238:errorcluster, "FP.State"=w236:T2)
                    n79 = case shown="\"Closed\"" w236 {
                      tunnel: [w244 w247] -> w241
                      tunnel: w238 -> [w243 w247]
                      tunnel: w237 -> [w242 _]
                      frame "Closed" {
                        n80 = invoke class="VI" method="FP.Open"(reference=w242, error in=w243, "Activate"=TRUE, "State"=T2."Standard") -> (error out=w244:errorcluster)  [unwired: 1 in, 4 out]
                      }
                      frame Default {
                      }
                    }
                  }
                  frame "Close" {
                    n81 = property class="VI"(reference=w250, error in=w252) -> (reference out=w249:refnum<vi>, error out=w251:errorcluster, "FP.State"=w248:T2)
                    n82 = case shown="Default" w248 {
                      tunnel: [w254 w257] -> w253
                      tunnel: w251 -> [w254 w256]
                      tunnel: w249 -> [_ w255]
                      frame "Invalid", "Closed" {
                      }
                      frame Default {
                        n83 = invoke class="VI" method="FP.Close"(reference=w255, error in=w256) -> (error out=w257:errorcluster)  [unwired: 1 in, 2 out]
                      }
                    }
                  }
                }
              }
              frame condition #1 {
              }
            }
            n84 = call <vilib>:"Add State(s) to Queue__jki_lib_state_machine.vi"("State(s) in (\"\")"=w231) -> ("States Out"=w230:string)  [unwired: 14 in]
          }
          frame "---------- Macro ----------" {
            # "Do not put any code in this frame.\n(It is a separator no-op. You can make a copy of this frame to create a new Macro frame)"
            n85 = call <vilib>:"Add State(s) to Queue__jki_lib_state_machine.vi"("State(s) in (\"\")"=w263) -> ("States Out"=w262:string)  [unwired: 14 in]
          }
          frame "Macro: Initialize" {
            w265 = "UI: Initialize\nMacro: Read UI Config\nAction: Open\nUI: Front Panel State >> Close\nMacro: Debug"  # UI: Initialize Macro: Read UI Config Action: Open UI: Front Panel State >> Close Macro: Debug
            # "Initialization Macro\n(This is called once, when the VI starts)"
            n86 = call <vilib>:"Add State(s) to Queue__jki_lib_state_machine.vi"("State(s) in Front (\"\")"="Data: Initialize\nInitialize Core Data\nEvents: Register", "State(s) in (\"\")"="Process: Sync", "State(s) at Back (\"\")"=w265) -> ("States Out"=w267:string)  [unwired: 12 in]
            n87 = call <vilib>:"Add State(s) to Queue__jki_lib_state_machine.vi"("State(s) in Front (\"\")"=w267, "State(s) in (\"\")"=w272) -> ("States Out"=w271:string)  [unwired: 13 in]
          }
          frame "Macro: Post Error Handling" {
            # "Clear Last Error?"
            n88 = Unbundle By Name(w274) -> ("Core.Last Error.remaining states"=w276:string, "Core.Shutdown?"=w277:bool)
            n89 = Unbundle By Name(w274) -> ("Core.Last Error.error"=w280:errorcluster)
            n90 = case shown="False" FALSE {
              tunnel: w280 -> [w288 _]
              tunnel: [w288 _] -> w279
              frame False {
              }
              frame True {
              }
            }
            n91 = case shown="False" w277 {
              tunnel: w276 -> [w285 w287]
              tunnel: [w285 w286] -> w273
              frame False {
                # "These are the remaining states (at the moment the error occured). States can be altered according to business logic."
                # "NOT SHUTTING DOWN"
              }
              frame True {
                # "Developer can decide to alter the states but should be aware that during the shutdown process, there are certain states that must be run for the SMO to properly shut itself (and this process) down. As such, one can add states to perform additional clean-ups, but should append the remaining state to be executed."
                # "SHUTTING DOWN"
                n92 = call <vilib>:"Add State(s) to Queue__jki_lib_state_machine.vi"("State(s) in (\"\")"=w287) -> ("States Out"=w286:string)  [unwired: 14 in]
              }
            }
            n93 = Bundle By Name(cluster=w274, "Core.Last Error.error"=w279) -> (w275:T10)
            n94 = call <vilib>:"Add State(s) to Queue__jki_lib_state_machine.vi"("State(s) in Front (\"\")"=w273, "State(s) in (\"\")"=w284) -> ("States Out"=w283:string)  [unwired: 13 in]
          }
          frame "Macro: Read UI Config" {
            # "Do not put any code in this frame.\n(It is a separator no-op. You can make a copy of this frame to create a new Macro frame)"
            n95 = call <vilib>:"Add State(s) to Queue__jki_lib_state_machine.vi"("State(s) in Front (\"\")"="Configuration: Initialize\nConfiguration: Read UI Config File\nUI: Update FP Controls" ("State(s) in Front (\"\")"), "State(s) in (\"\")"=w294) -> ("States Out"=w293:string)  [unwired: 13 in]
          }
          frame "Macro: Write UI Config" {
            # "Do not put any code in this frame.\n(It is a separator no-op. You can make a copy of this frame to create a new Macro frame)"
            n96 = call <vilib>:"Add State(s) to Queue__jki_lib_state_machine.vi"("State(s) in Front (\"\")"="Data: Set UI Cluster\nConfiguration: Write UI Config File" ("State(s) in Front (\"\")"), "State(s) in (\"\")"=w300) -> ("States Out"=w299:string)  [unwired: 13 in]
          }
          frame "Macro: Debug" {
            n97 = Unbundle By Name(w302) -> ("UI Behavior"=w304:string)
            n98 = Format Into String(format string="Data: Debug\nUI: Front Panel State >> %s\n//UI: Wait" ("State(s) in Front (\"\")"), w304) -> (resulting string=w301:string)  [unwired: 2 in, 1 out]
            n99 = call <vilib>:"Add State(s) to Queue__jki_lib_state_machine.vi"("State(s) in Front (\"\")"=w301, "State(s) in (\"\")"=w308) -> ("States Out"=w307:string)  [unwired: 13 in]
          }
          frame "Macro: Exit" {
            # "Exit Macro\n(This is called once, when the VI exits)"
            n100 = Unbundle By Name(w312) -> ("Core.Close Panel on Exit?"=w310:bool)
            n101 = Select(t="UI: Front Panel State >> Close", s=w310, f="" ("Empty String Constant")) -> (s? t:f=w319:string)
            n102 = call <vilib>:"Add State(s) to Queue__jki_lib_state_machine.vi"("State(s) in Front (\"\")"="Data: Cleanup\nEvents: Unregister\nProcess: Self Terminate", "State(s) in (\"\")"="Process: Sync", "State(s) at Back (\"\")"="Exit") -> ("States Out"=w314:string)  [unwired: 12 in]
            n103 = call <vilib>:"Add State(s) to Queue__jki_lib_state_machine.vi"("State(s) in Front (\"\")"="Action: Close\nMacro: Write UI Config", "State(s) in (\"\")"=w319, "State(s) at Back (\"\")"=w314) -> ("States Out"=w318:string)  [unwired: 12 in]
            n104 = call <vilib>:"Add State(s) to Queue__jki_lib_state_machine.vi"("State(s) in Front (\"\")"=w318, "State(s) in (\"\")"=w323) -> ("States Out"=w322:string)  [unwired: 13 in]
          }
          frame "---------- Process ----------" {
            # "Template Separator\n(You can make a copy of, or modify, this frame)"
            n105 = call <vilib>:"Add State(s) to Queue__jki_lib_state_machine.vi"("State(s) in (\"\")"=w328) -> ("States Out"=w327:string)  [unwired: 14 in]
          }
          frame "Process: Sync" {
            n106 = Unbundle By Name(w336) -> ("Instrument UI"=w332:refnum<class "Inst UI.Transport.lvclass">)
            n107 = call <vilib>:"WaitOnProcessSync.vi"("error in (no error)"=w331, "SMO"=w332) -> ("error out"=w330:errorcluster, "Don't run?"=w335:bool)  [unwired: 7 in, 1 out]
            n108 = Select(t="Data: Cleanup\nEvents: Unregister\nExit", s=w335, f="" ("Empty String Constant")) -> (s? t:f=w329:string)
            n109 = call <vilib>:"Add State(s) to Queue__jki_lib_state_machine.vi"("State(s) in Front (\"\")"=w329, "State(s) in (\"\")"=w339) -> ("States Out"=w338:string)  [unwired: 13 in]
          }
          frame "Process: Self Terminate" {
            n110 = Unbundle By Name(w341) -> ("Instrument UI"=w340:refnum<class "Inst UI.Transport.lvclass">)
            n111 = call <vilib>:"SelfTerminate.vi"("error in (no error)"=w343, "SMO in"=w340) -> ("error out"=w342:errorcluster)  [unwired: 8 in, 1 out]
            n112 = call <vilib>:"Add State(s) to Queue__jki_lib_state_machine.vi"("State(s) in (\"\")"=w346) -> ("States Out"=w345:string)  [unwired: 14 in]
          }
          frame "---------- Events ----------" {
            # "Template Separator\n(You can make a copy of, or modify, this frame)"
            n113 = call <vilib>:"Add State(s) to Queue__jki_lib_state_machine.vi"("State(s) in (\"\")"=w351) -> ("States Out"=w350:string)  [unwired: 14 in]
          }
          frame "Events: Register" {
            # "Expand to add\nmore events"
            # "Base Class Protected Events"
            n114 = Unbundle By Name(w362) -> ("Instrument UI"=w353:refnum<class "Inst UI.Transport.lvclass">, "Instrument"=w352:refnum<class "Inst.Transport.lvclass">)
            n115 = call <vilib>:"GetProtectedEvents.vi"("SMO"=w353) -> ("error out"=w356:errorcluster, "SMO Protected Events"=w360:T13)  [unwired: 8 in, 1 out]
            n116 = call <userlib>:"Instrument.GetPublicEvents.vi"("Instrument"=w352) -> ("error out"=w354:errorcluster, "Instrument Public Events"=w355:T14)  [unwired: 8 in, 1 out]
            n117 = register-events(w360, w355) -> (reference out=w361:refnum<event-registration>, error out=w358:errorcluster)  [unwired: 2 in]
            n118 = Merge Errors(w354, w359, w358, w356) -> (w357:errorcluster)
            n119 = call <vilib>:"Add State(s) to Queue__jki_lib_state_machine.vi"("State(s) in (\"\")"=w364) -> ("States Out"=w363:string)  [unwired: 14 in]
          }
          frame "Events: Unregister" {
            n120 = Unregister For Events(event registration refnum=w367, error in=w366) -> (error out=w365:errorcluster)
            n121 = call <vilib>:"Add State(s) to Queue__jki_lib_state_machine.vi"("State(s) in (\"\")"=w370) -> ("States Out"=w369:string)  [unwired: 14 in]
          }
          frame "---------- Configuration ----------" {
            # "Do not put any code in this frame.\n(It is a separator no-op. You can make a copy of this frame to create a new UI frame)"
            n122 = call <vilib>:"Add State(s) to Queue__jki_lib_state_machine.vi"("State(s) in (\"\")"=w375) -> ("States Out"=w374:string)  [unwired: 14 in]
          }
          frame "Configuration: Initialize" {
            # "Do not put any code in this frame.\n(It is a separator no-op. You can make a copy of this frame to create a new UI frame)"
            n123 = Unbundle By Name(w383) -> ("Configuration"=w381:refnum<class "Configuration.lvclass">, "Instrument"=w382:refnum<class "Inst.Transport.lvclass">)
            n124 = call <vilib>:"GetName.vi"("error in (no error)"=w385, "SMO"=w382) -> ("error out"=w384:errorcluster, "Name"=w386:string)  [unwired: 6 in, 2 out]
            n125 = call <userlib>:"Default Path.vi"("error in (no error)"=w384, "Folder Name [Application Name]"=w386, "Configuration in"=w381) -> ("error out"=w377:errorcluster, "Configuration out"=w380:refnum<class "Configuration.lvclass">)  [unwired: 7 in]
            n126 = call <userlib>:"Write Section.vi"("error in (no error)"=w377, "Section"="UI", "Configuration in"=w380) -> ("error out"=w376:errorcluster, "Configuration out"=w379:refnum<class "Configuration.lvclass">)  [unwired: 7 in]
            n127 = Bundle By Name(cluster=w383, "Configuration"=w379) -> (w387:T10)
            n128 = call <vilib>:"Add State(s) to Queue__jki_lib_state_machine.vi"("State(s) in (\"\")"=w390) -> ("States Out"=w389:string)  [unwired: 14 in]
          }
          frame "Configuration: Write UI Config File" {
            # "Do not put any code in this frame.\n(It is a separator no-op. You can make a copy of this frame to create a new Data frame)"
            n129 = Unbundle By Name(w395) -> ("Configuration"=w392:refnum<class "Configuration.lvclass">, "UI Cluster"=w394:T9)
            n130 = call <userlib>:"Write Configuration.vi"("error in (no error)"=w391, "Variant"=w394, "Configuration in"=w392) -> ("error out"=w393:errorcluster)  [unwired: 7 in, 1 out]
            n131 = call <vilib>:"Add State(s) to Queue__jki_lib_state_machine.vi"("State(s) in (\"\")"=w398) -> ("States Out"=w397:string)  [unwired: 14 in]
          }
          frame "Configuration: Read UI Config File" {
            # "Do not put any code in this frame.\n(It is a separator no-op. You can make a copy of this frame to create a new UI frame)"
            n132 = Unbundle By Name(w401) -> ("UI Cluster"=w404:T9, "Configuration"=w407:refnum<class "Configuration.lvclass">)
            n133 = call <userlib>:"Read Configuration.vi"("INI Fomatted Cluster Type"=w404, "error in (no error)"=w403, "Configuration in"=w407) -> ("error out"=w406:errorcluster, "Configuration"=w405:variant)  [unwired: 6 in, 1 out]
            n134 = Variant To Data(error in=w406, type=w404, Variant=w405) -> (data=w400:T9, error out=w402:errorcluster)
            n135 = Bundle By Name(cluster=w401, "UI Cluster"=w400) -> (w399:T10)
            n136 = call <vilib>:"Add State(s) to Queue__jki_lib_state_machine.vi"("State(s) in (\"\")"=w410) -> ("States Out"=w409:string)  [unwired: 14 in]
          }
          frame "---------- Action ----------" {
            n137 = Unbundle By Name(w413) -> ("Instrument UI"=w411:refnum<class "Inst UI.Transport.lvclass">)
            n138 = Bundle By Name(cluster=w413, "Instrument UI"=w411) -> (w412:T10)
            n139 = call <vilib>:"Add State(s) to Queue__jki_lib_state_machine.vi"("State(s) in (\"\")"=w417) -> ("States Out"=w416:string)  [unwired: 14 in]
          }
          frame "Action: Notify UI Closed" {
            # "Notify that the UI has been closed"
            n140 = Unbundle By Name(w418) -> ("Instrument UI"=w421:refnum<class "Inst UI.Transport.lvclass">)
            n141 = call <vilib>:"Hide.vi"("error in (no error)"=w420, "SMO.UI"=w421) -> ("error out"=w419:errorcluster)  [unwired: 8 in, 1 out]
            n142 = call <vilib>:"Add State(s) to Queue__jki_lib_state_machine.vi"("State(s) in (\"\")"=w424) -> ("States Out"=w423:string)  [unwired: 14 in]
          }
          frame "Action: getAll" {
            n143 = Unbundle By Name(w433) -> ("getAll"=w426:T8, "Instrument"=w427:refnum<class "Inst.Transport.lvclass">)
            n144 = call <userlib>:"getAll.vi"("error in (no error)"=w425, "Instrument in"=w427) -> ("error out"=w432:errorcluster, "getAll"=w428:variant, "Instrument out"=w429:refnum<class "Inst.Transport.lvclass">)  [unwired: 7 in]
            n145 = call "JSON to LVtype.vim"("type"=w426, "error in (no error)"=w432, "JSON Data in"=w428) -> ("error out"=w431:errorcluster, "Data out"=w430:T8)  [unwired: 7 in]
            n146 = Bundle By Name(cluster=w433, "Instrument"=w429, "getAll"=w430) -> (w434:T10)
            n147 = call <vilib>:"Add State(s) to Queue__jki_lib_state_machine.vi"("State(s) in Front (\"\")"="" ("State(s) in Front (\"\")"), "State(s) in (\"\")"=w438) -> ("States Out"=w437:string)  [unwired: 13 in]
          }
          frame "Action: Open" {
            # "local/remote?"
            n148 = Unbundle By Name(w442) -> ("Instrument"=w440:refnum<class "Inst.Transport.lvclass">)
            n149 = call-dynamic "Open.vi"("error in (no error)"=w439, "Inst.Transport in"=w440) -> ("error out"=w445:errorcluster, "Inst.Transport out"=w441:refnum<class "Inst.Transport.lvclass">)  [unwired: 8 in]
            n150 = Bundle By Name(cluster=w442, "Instrument"=w441) -> (w443:T10)
            n151 = call <vilib>:"Add State(s) to Queue__jki_lib_state_machine.vi"("State(s) in Front (\"\")"="" ("State(s) in Front (\"\")"), "State(s) in (\"\")"=w448) -> ("States Out"=w447:string)  [unwired: 13 in]
          }
          frame "Action: Close" {
            n152 = Unbundle By Name(w450) -> ("Instrument"=w453:refnum<class "Inst.Transport.lvclass">)
            n153 = call-dynamic "Close.vi"("error in (no error)"=w451, "Inst.Transport in"=w453) -> ("error out"=w455:errorcluster, "Inst.Transport out"=w449:refnum<class "Inst.Transport.lvclass">)  [unwired: 8 in]
            n154 = Bundle By Name(cluster=w450, "Instrument"=w449) -> (w452:T10)
            n155 = call <vilib>:"Add State(s) to Queue__jki_lib_state_machine.vi"("State(s) in Front (\"\")"="" ("State(s) in Front (\"\")"), "State(s) in (\"\")"=w458) -> ("States Out"=w457:string)  [unwired: 13 in]
          }
        }
      }
    }
    frame Error {
    }
  }
  n156 = call-parent "Process.vi"("error in"=w5, "Instrument UI in"=w4) -> ("error out"=w2:errorcluster, "Instrument UI out"=→"Instrument UI.Transport out":refnum<class "Inst UI.Transport.lvclass">)  [unwired: 8 in]
  n157 = Merge Errors(w2, w1) -> (→"error out":errorcluster)
